vi "classify error.vi"(8 "error to classify":errorcluster, 11 "Tagbus PID Module runtime in":refnum<class "Tagbus PID Module runtime.lvclass">) -> (0 "classified error":errorcluster, 2 "error classification":T1, 3 "Tagbus PID Module runtime out":refnum<class "Tagbus PID Module runtime.lvclass">)   [LabVIEW 2014, in "Tagbus PID Module runtime.lvclass"]
doc: "Allows a module to classify an error generated at any point during execution. This <b>error classification</b> can then be used by calling code to determine if execution can continue. In addition, this function can be used to allow a component to clear an error, convert an error to a warning, or attempt to recover from an error. Recovery may be attempted only if <b>attempt recovery?</b> is true."
uses:
  Tagbus PID Module runtime.lvclass
  <vilib>/NI/Tag Bus Module Framework/runtime/error classification.ctl
  <vilib>/NI/Tag Bus Module Framework/runtime/TBM module execution interface.lvclass
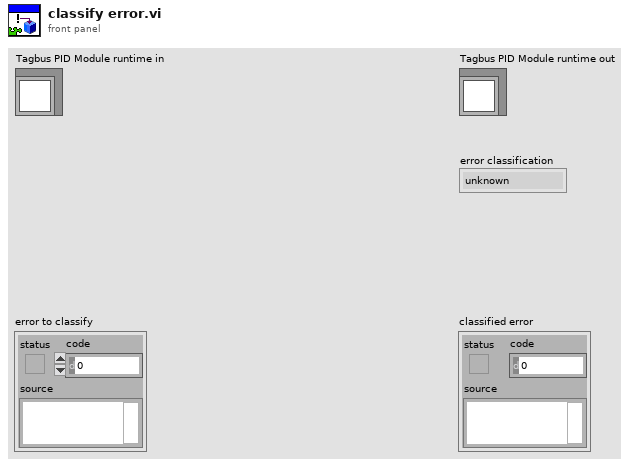
[diagram p1: front panel]
types:
  T1 = typedef "TBM module execution interface.lvclass/error classification.ctl" = enum16{"unknown", "none", "trivial", "recoverable", "critical"}
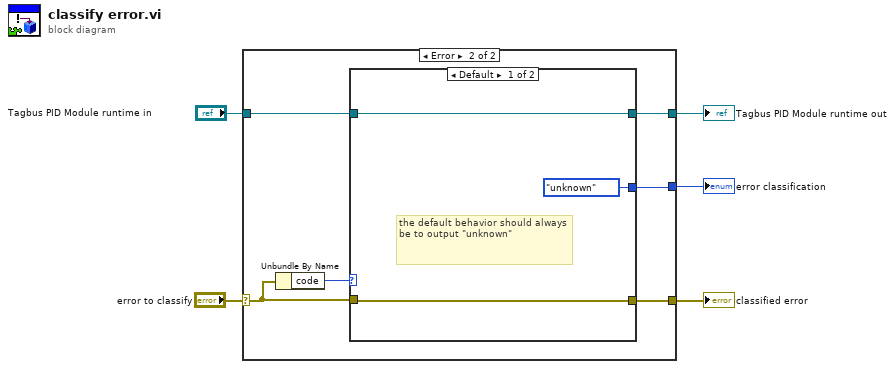
[diagram p0: block diagram]
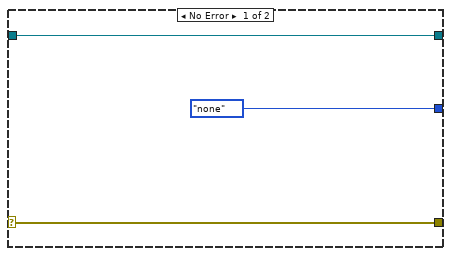
[diagram p2: hidden frame]
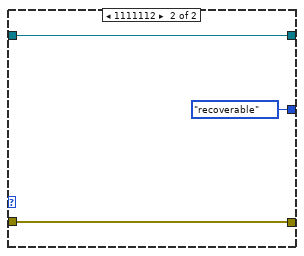
[diagram p3: hidden frame]
diagram:
  n1 = case shown="Error" "error to classify" {
    selector: "error to classify" -> [w7 w13]
    tunnel: [w8 w9] -> w4
    tunnel: "Tagbus PID Module runtime in" -> [w8 w10]
    tunnel: [w7 w12] -> w2
    tunnel: [error_classification."none" ("error classification") w11] -> w1
    frame No Error {
    }
    frame Error {
      n2 = Unbundle By Name(w13) -> ("code"=w14:i32)
      n3 = case shown="Default" w14 {
        tunnel: w13 -> [w15 w20]
        tunnel: [w15 w20] -> w12
        tunnel: [error_classification."unknown" ("error classification") error_classification."recoverable" ("error classification")] -> w11
        tunnel: w10 -> [w16 w18]
        tunnel: [w16 w18] -> w9
        frame Default {
          # "the default behavior should always be to output \"unknown\""
        }
        frame 1111112 {
        }
      }
    }
  }
  "Tagbus PID Module runtime out" <- w4
  "error classification" <- w1
  "classified error" <- w2
